vi "Neutral_48ch_PB_write.vi"(8 "Error In":errorcluster, 10 "48ch_pb_array":T2 {"Label and Instructions"."Instruct Data" format="%#.2p"; "Label and Instructions"."Op Code" items=["Continue", "Stop", "Loop", "End Loop", "JSR", "RTS", "Go To", "Long Delay", "Wait"]; "Label and Instructions"."Time (s)" min=5e-08 format="%.2p"}) -> (0 "error out":errorcluster)   [LabVIEW 2016]
uses:
  Controls/PulseBlaster/48ch_pb_array.ctl
  Controls/PulseBlaster/48ch_single_timing_column_condensed.ctl
  Controls/ExperimentParameters/experimentalvariables.ctl
panel:
  in  "Experimental Variables":T1={"Pixel Size before binning (µm)"=6.0, "Imaging Wavelength (m)"=4.61e-07, "Isotope"=87, "1P1 Linewidth (MHz)"=30.5, "Imaging Detuning (MHz)"=0.0, "Software Bin Size"=1, "Exp. Trigger ON time (ms)"=50.0, "Path to spinapi.dll"=path "C:/SpinCore/SpinAPI/lib32/spinapi.dll", "PB clock_freq (MHz)"=100.0} {"Software Bin Size" items=["1"=1, "2"=2, "3"=3, "4"=4, "5"=5, "6"=6, "7"=7, "8"=8]; "Isotope" min=84 max=88; "Imaging Wavelength (m)" format="%#_6p"}
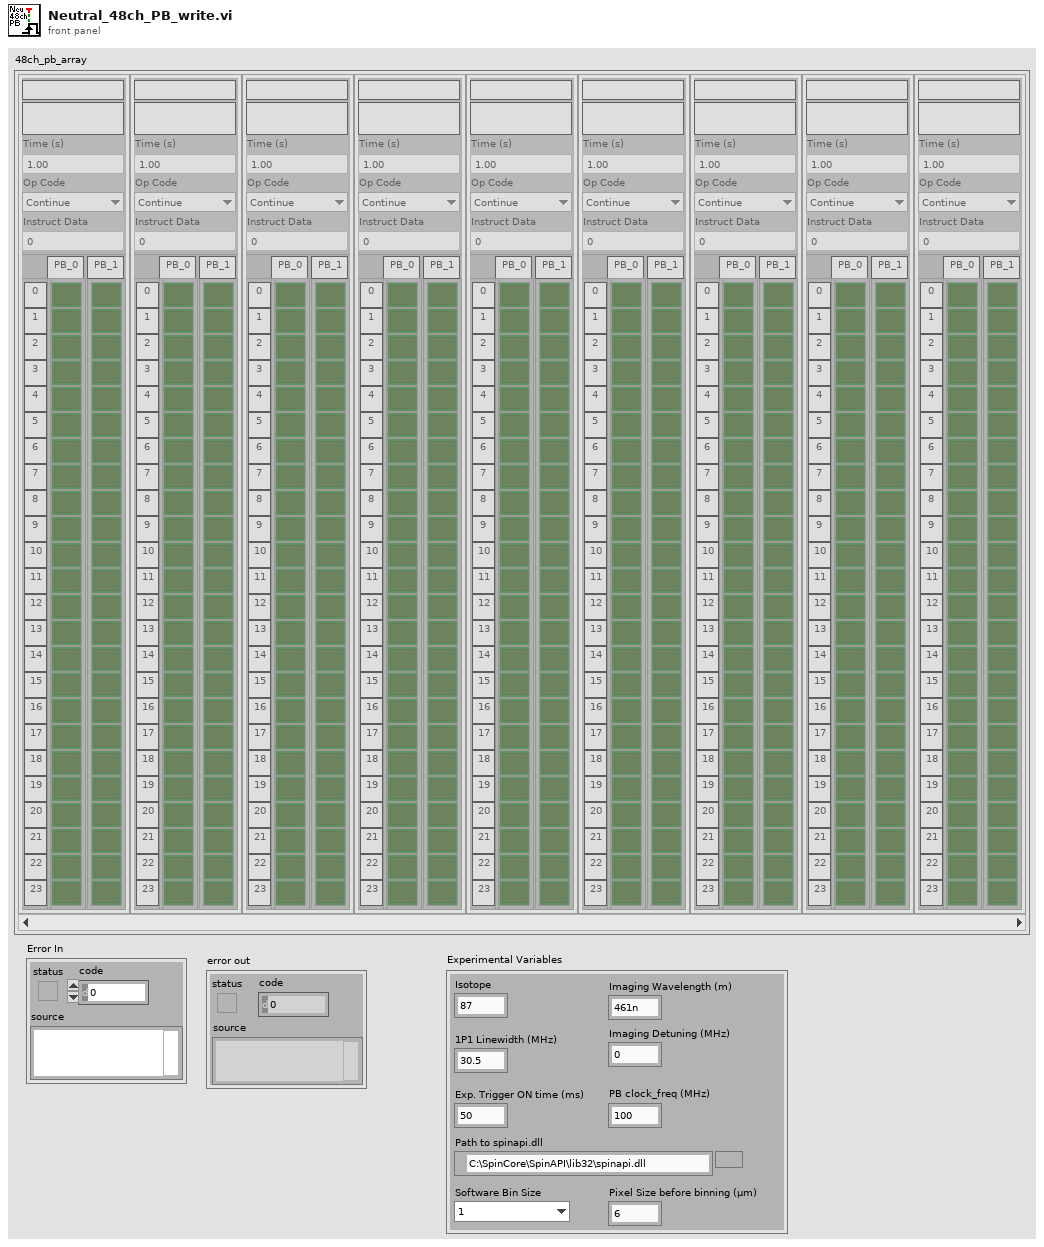
[diagram p1: front panel]
types:
  T1 = typedef "experimentalvariables.ctl" = cluster{"Pixel Size before binning (µm)":dbl, "Imaging Wavelength (m)":dbl, "Isotope":i32, "1P1 Linewidth (MHz)":dbl, "Imaging Detuning (MHz)":dbl, "Software Bin Size":u16, "Exp. Trigger ON time (ms)":dbl, "Path to spinapi.dll":path, "PB clock_freq (MHz)":dbl}
  T2 = typedef "48ch_pb_array.ctl" = T3[]
  T3 = typedef "48ch_single_timing_column_condensed.ctl" = cluster{"Label and Instructions":cluster{"Column Number":string, "Comments":string, "Time (s)        ":dbl, "Op Code":i32, "Instruct Data":i32}, "PB_1_Bools":bool[], "Column Number":string, "Column Number 2":string, "PB_0_Bools":bool[], "Ch_Labels":string[]}
  T4 = typedef "24ch_pb_array.ctl" = T5[]
  T5 = typedef "24ch_single_timing_column.ctl" = cluster{"Instruct Data":i32, "Op Code":i32, "Flags":bool[], "Comments":string, "Time (s)":dbl}
  T6 = enum16{"Pulse Program", "Frequency Registers", "TX Phase Registers", "RX Phase Registers"}
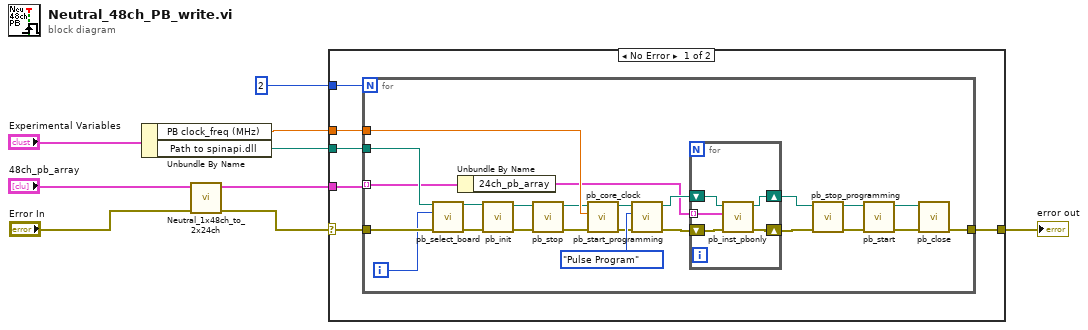
[diagram p0: block diagram]
diagram:
  n1 = Unbundle By Name("Experimental Variables") -> ("PB clock_freq (MHz)"=w2:dbl, "Path to spinapi.dll"=w3:path)
  n2 = call "Neutral_1x48ch_to_2x24ch.vi"("Error In"="Error In", "48ch_pb_array"="48ch_pb_array") -> ("error out"=w5:errorcluster, "1D_array_of_24ch_pb_array"=w6:cluster{"24ch_pb_array":T4}[])  [unwired: 8 in]
  n3 = case shown="No Error" w5 {
    selector: w5 -> [w10 w45]
    tunnel: 2 -> [w15 _]
    tunnel: w3 -> [w14 _]
    tunnel: w2 -> [w13 _]
    tunnel: [w12 w45] -> w1
    tunnel: w6 -> [w11 _]
    frame No Error {
      n4 = for {
        N: w15 -> [_]
        tunnel: w10 -> [w39]
        tunnel: w14 -> [w29]
        tunnel: w13 -> [w27]
        tunnel: [w22] -> w12
        tunnel: w11 -> [w17] mode=indexing
        i -> [w38]
        n5 = call "pb_select_board.vi"("error in (no error)"=w39, "board_num"=w38, "path in"=w29) -> ("error out"=w30:errorcluster, "path out"=w28:path)  [unwired: 7 out]
        n6 = Unbundle By Name(w17) -> ("24ch_pb_array"=w16:T4)
        n7 = call "pb_init.vi"("error in (no error)"=w30, "path in"=w28) -> ("error out"=w20:errorcluster, "path out"=w21:path)  [unwired: 2 in, 6 out]
        n8 = call "pb_stop.vi"("error in (no error)"=w20, "path in"=w21) -> ("error out"=w19:errorcluster, "path out"=w18:path)  [unwired: 8 out]
        n9 = call "pb_core_clock.vi"("error in (no error)"=w19, "clock_freq (MHz)"=w27, "path in"=w18) -> ("error out"=w31:errorcluster, "path out"=w32:path)  [unwired: 7 in]
        n10 = call "pb_start_programming.vi"("error in (no error)"=w31, "Device"=T6."Pulse Program", "path in"=w32) -> ("error out"=w34:errorcluster, "path out"=w37:path)  [unwired: 1 in, 6 out]
        n11 = for {
          tunnel: w16 -> [w40] mode=indexing
          shift-right: [w43] -> w36
          shift-left: w37 -> [w44]
          shift-right: [w41] -> w33
          shift-left: w34 -> [w42]
          n12 = call "pb_inst_pbonly.vi"("error in (no error)"=w42, "PB Instruction"=w40, "path in"=w44) -> ("error out"=w41:errorcluster, "path out"=w43:path)  [unwired: 2 in, 5 out]
        }
        n13 = call "pb_stop_programming.vi"("error in (no error)"=w33, "path in"=w36) -> ("error out"=w24:errorcluster, "path out"=w26:path)  [unwired: 1 in, 7 out]
        n14 = call "pb_start.vi"("error in (no error)"=w24, "path in"=w26) -> ("error out"=w23:errorcluster, "path out"=w25:path)  [unwired: 1 in, 7 out]
        n15 = call "pb_close.vi"("error in (no error)"=w23, "path in"=w25) -> ("error out"=w22:errorcluster)  [unwired: 9 out]
      }
    }
    frame Error {
    }
  }
  "error out" <- w1
